vi "Find Monkey Containing Variable in its Job.vi"(4 "Monkeys":T1, 5 "Variable":string, 6 "Monkey Job Statement":string) -> (0 "Monkey having Variable in its Job":string, 1 "Variable is in Right Monkey's Job ?":bool, 2 "Operator":string, 3 "Monkey not having Variable in its Job":string)   [LabVIEW 2020, in "AoC 2022.lvlib"]
uses:
  AoC 2022.lvlib
  Day 11 - Monkey in the Middle/private/Monkeys.ctl
  Day 11 - Monkey in the Middle/private/Monkey.ctl
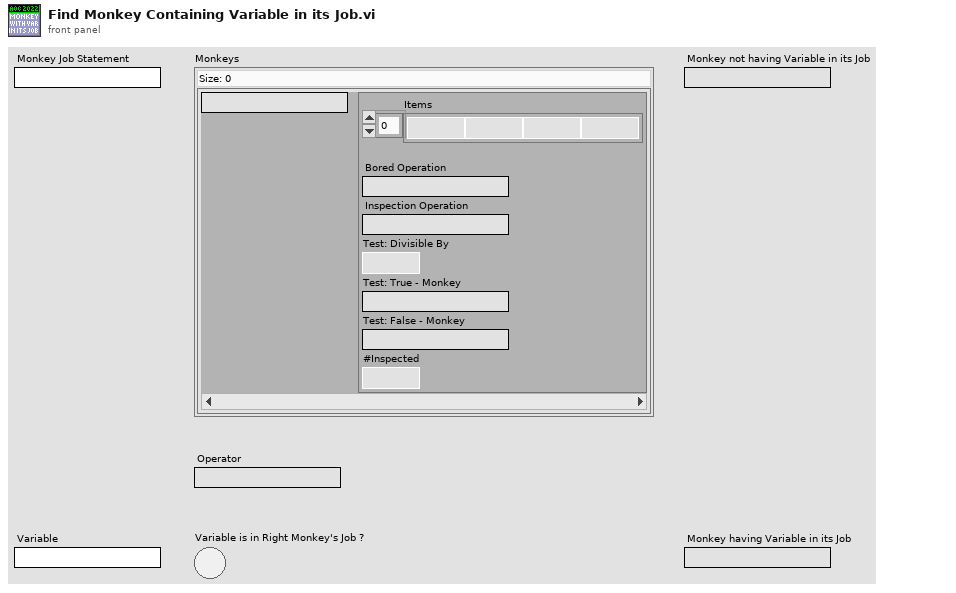
[diagram p1: front panel]
types:
  T1 = typedef "AoC 2022.lvlib/Monkeys.ctl" = map{string, T2}
  T2 = typedef "AoC 2022.lvlib/Monkey.ctl" = cluster{"Items":u64[], "Bored Operation":string, "Inspection Operation":string, "Test: Divisible By":u64, "Test: True - Monkey":string, "Test: False - Monkey":string, "#Inspected":i32}
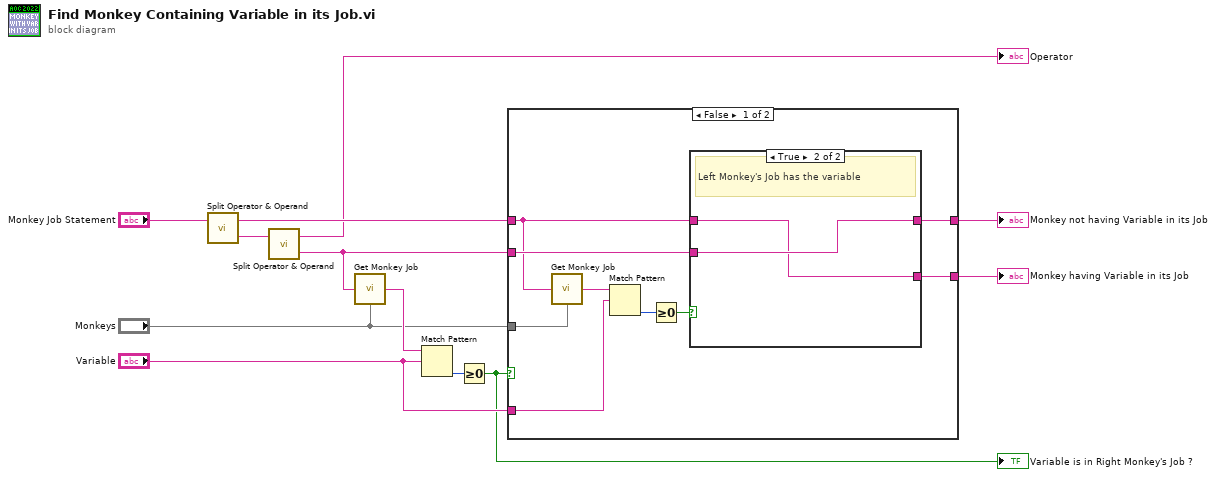
[diagram p0: block diagram]
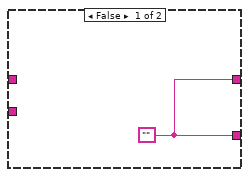
[diagram p2: hidden frame]
diagram:
  n1 = call "Split Operator & Operand.vi"("Operation"="Monkey Job Statement") -> ("Operand"=w7:string, "Operator"=w9:string)  [unwired: 1 in]
  n2 = call "Split Operator & Operand.vi"("Operation"=w7) -> ("Operand"=w10:string, "Operator"=→"Operator":string)  [unwired: 1 in]
  n3 = call "Get Monkey Job.vi"("Monkey"=w10, "Monkeys"="Monkeys") -> ("Monkey Job"=w8:string)
  n4 = Match Pattern(string=w8, regular expression="Variable") -> (offset past match=w5:i32)  [unwired: 1 in, 3 out]
  n5 = Greater Or Equal To 0?(x=w5) -> (x >= 0?=w1:bool)
  "Variable is in Right Monkey's Job ?" <- w1
  n6 = case shown="False" w1 {
    tunnel: w9 -> [w13 w26]
    tunnel: w10 -> [w15 w25]
    tunnel: [w16 w26] -> w11
    tunnel: [w14 w25] -> w12
    tunnel: "Monkeys" -> [w21 _]
    tunnel: "Variable" -> [w18 _]
    frame False {
      n7 = call "Get Monkey Job.vi"("Monkey"=w13, "Monkeys"=w21) -> ("Monkey Job"=w19:string)
      n8 = Match Pattern(string=w19, regular expression=w18) -> (offset past match=w20:i32)  [unwired: 1 in, 3 out]
      n9 = Greater Or Equal To 0?(x=w20) -> (x >= 0?=w17:bool)
      n10 = case shown="True" w17 {
        tunnel: [w22 w24] -> w16
        tunnel: w15 -> [_ w24]
        tunnel: [w22 w23] -> w14
        tunnel: w13 -> [_ w23]
        frame False {
          w22 = ""
        }
        frame True {
          # "Left Monkey's Job has the variable"
        }
      }
    }
    frame True {
      # "Right Monkey's Job has the variable"
    }
  }
  "Monkey having Variable in its Job" <- w12
  "Monkey not having Variable in its Job" <- w11
